vi "Main.Load 986x Bitfile.vi"(8 "error in (no error)":errorcluster, 11 "FPGA Settings":T1) -> (0 "error out":errorcluster, 2 "FPGA Session":u32)   [LabVIEW 2023, in "J1939 Addon Engine.lvlib"]
uses:
  J1939 Addon Engine.lvlib
  Addon Shared/Types/SysDef FPGA Settings.ctl
  Addon Shared/J1939 Addon Shared.lvlib
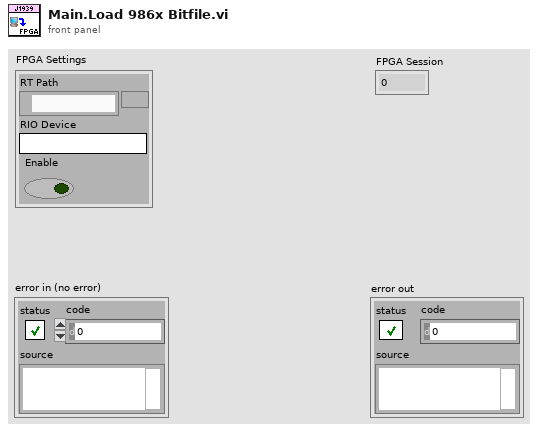
[diagram p1: front panel]
types:
  T1 = typedef "J1939 Addon Shared.lvlib/SysDef FPGA Settings.ctl" = cluster{"RT Path":path, "RIO Device":string, "Enable":bool}
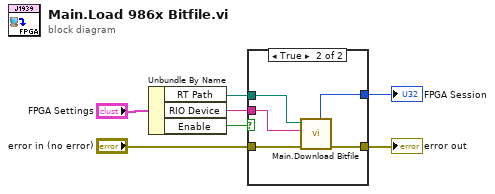
[diagram p0: block diagram]
diagram:
  n1 = Unbundle By Name("FPGA Settings") -> ("RT Path"=w4:path, "RIO Device"=w3:string, "Enable"=w2:bool)
  n2 = case shown="True" w2 {
    tunnel: "error in (no error)" -> [w8 w9]
    tunnel: [w8 w13] -> w7
    tunnel: [_ w12] -> w6
    tunnel: w4 -> [_ w11]
    tunnel: w3 -> [_ w10]
    frame False {
    }
    frame True {
      n3 = call "Main.Download Bitfile.vi"("error in (no error)"=w9, "RIO Device"=w10, "path"=w11) -> ("error out"=w13:errorcluster, "FPGA Session"=w12:u32)  [unwired: 7 in]
    }
  }
  "error out" <- w7
  "FPGA Session" <- w6
